vi "Machine Setting - Sensor Parse Read Data (SubVI).vi"(11 "Sensor":T1) -> (3 "Array":string[](array[string]))   [LabVIEW 2019]
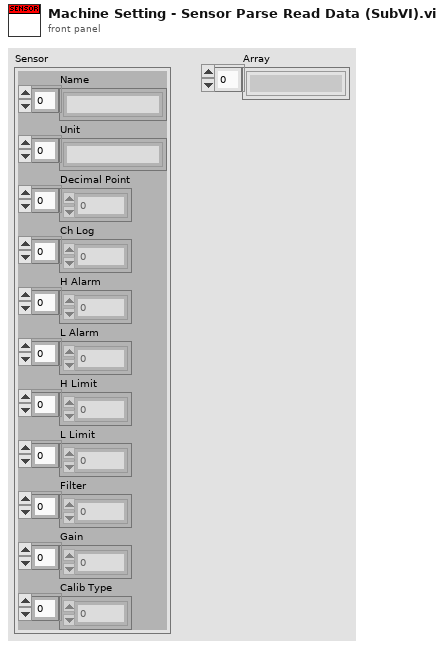
[diagram p1: front panel]
types:
  T1 = cluster{"Name":string[], "Unit":string[], "Decimal Point":u8[], "Ch Log":u8[], "H Alarm":u8[], "L Alarm":u8[], "H Limit":sgl[], "L Limit":sgl[], "Filter":u8[], "Gain":u8[], "Calib Type":u32[]}
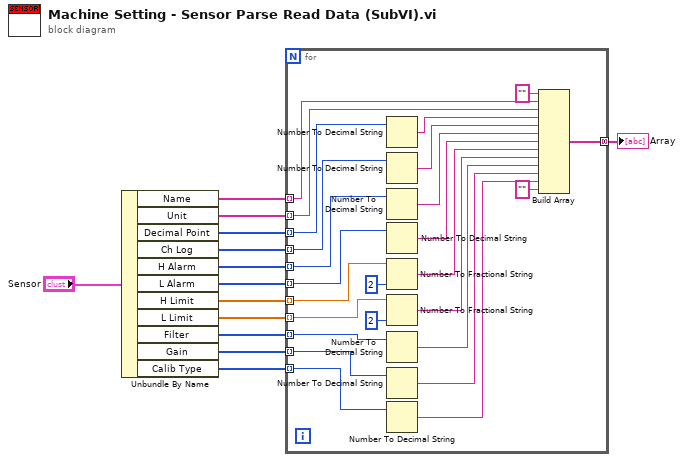
[diagram p0: block diagram]
diagram:
  n1 = Unbundle By Name("Sensor") -> ("Name"=w1:string[], "Unit"=w2:string[], "Decimal Point"=w4:u8[], "Ch Log"=w5:u8[], "H Alarm"=w6:u8[], "L Alarm"=w7:u8[], "H Limit"=w8:sgl[], "L Limit"=w9:sgl[], "Filter"=w10:u8[], "Gain"=w11:u8[], "Calib Type"=w12:u32[])
  n2 = for {
    tunnel: w1 -> [w38] mode=indexing
    tunnel: w2 -> [w37] mode=indexing
    tunnel: w4 -> [w36] mode=indexing
    tunnel: w5 -> [w35] mode=indexing
    tunnel: w6 -> [w34] mode=indexing
    tunnel: w7 -> [w33] mode=indexing
    tunnel: w8 -> [w32] mode=indexing
    tunnel: w9 -> [w30] mode=indexing
    tunnel: w10 -> [w28] mode=indexing
    tunnel: w11 -> [w27] mode=indexing
    tunnel: w12 -> [w26] mode=indexing
    tunnel: [w14] -> w13 mode=concatenating
    n3 = Number To Decimal String(number=w36) -> (decimal integer string=w25:string)  [unwired: 1 in]
    n4 = Number To Decimal String(number=w35) -> (decimal integer string=w24:string)  [unwired: 1 in]
    n5 = Number To Decimal String(number=w34) -> (decimal integer string=w23:string)  [unwired: 1 in]
    n6 = Number To Decimal String(number=w33) -> (decimal integer string=w22:string)  [unwired: 1 in]
    n7 = Number To Fractional String(number=w32, precision (6)=i16 2) -> (F-format string=w21:string)  [unwired: 2 in]
    n8 = Number To Fractional String(number=w30, precision (6)=i16 2) -> (F-format string=w20:string)  [unwired: 2 in]
    n9 = Number To Decimal String(number=w28) -> (decimal integer string=w19:string)  [unwired: 1 in]
    n10 = Number To Decimal String(number=w27) -> (decimal integer string=w18:string)  [unwired: 1 in]
    n11 = Number To Decimal String(number=w26) -> (decimal integer string=w17:string)  [unwired: 1 in]
    n12 = Build Array("" ("element"), w38, w37, w25, w24, w23, w22, w21, w20, w19, w18, w17, "" ("element")) -> (w14:string[])
  }
  "Array" <- w13
